vi "GB Situation.vi"(0 "GB defects":dbl, 5 "def type":i8, 7 "thr1":dbl, 9 "thr2":dbl) -> (6 "GB sit":i8)   [LabVIEW 2019]
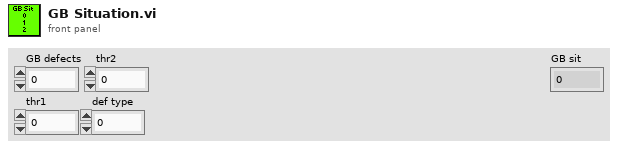
[diagram p1: front panel]
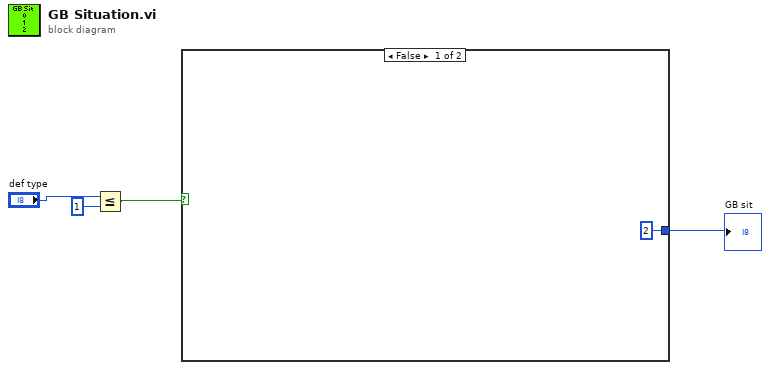
[diagram p0: block diagram]
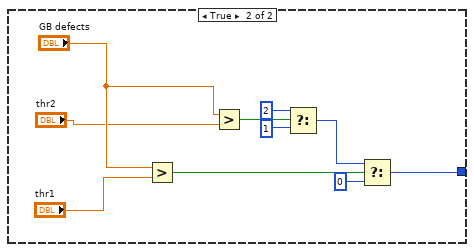
[diagram p2: hidden frame]
diagram:
  n1 = Less Or Equal?(x="def type", y=i8 1) -> (x <= y?=w2:bool)
  n2 = case shown="False" w2 {
    tunnel: [i8 2 ("f") w6] -> w1
    frame False {
    }
    frame True {
      n3 = Greater?(x="GB defects", y="thr1") -> (0:w14:bool)
      n4 = Greater?(x="GB defects", y="thr2") -> (0:w11:bool)
      n5 = Select(t=i8 2, s=w11, f=i8 1 ("t")) -> (s? t:f=w8:i8)
      n6 = Select(t=w8, s=w14, f=i8 0) -> (s? t:f=w6:i8)
    }
  }
  "GB sit" <- w1
